vi "Mischer_flowmeter_readout.vi"() -> (0 "Flow \n[µmol/sec He-3*(100]":dbl format="%#.1p")   [LabVIEW 2018]
uses:
  Global/Global Variables/Data_Display_global.vi
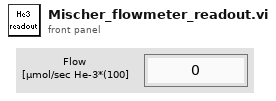
[diagram p1: front panel]
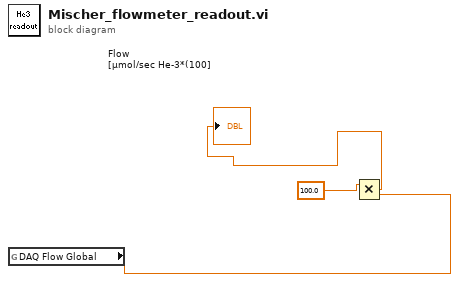
[diagram p0: block diagram]
diagram:
  n1 = global read "Data_Display_global.vi" "DAQ Flow Global"() -> (w1:dbl)
  n2 = Multiply(x=100.0, y=w1) -> (x*y=→"Flow \n[µmol/sec He-3*(100]":dbl)
